vi "prepare droplet.vi"(3 "channel":i8) -> ()   [LabVIEW 2023]
panel:
  out "sum":i32
  out "entry":i32
  out "stock array":string[](array[string])
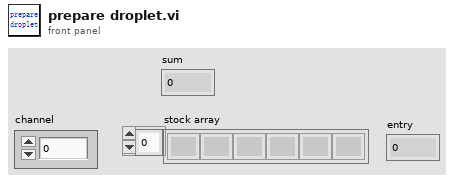
[diagram p1: front panel]
types:
  T1 = enum16{"Initialize", "Absolute Position", "Relative Pickup", "Relative Dispense", "Swich valve", "Bypass"}
  T2 = enum16{"check", "scan", "index", "read", "add", "write"}
  T3 = enum16{"plate1", "plate2", "plate3", "rinse", "seat"}
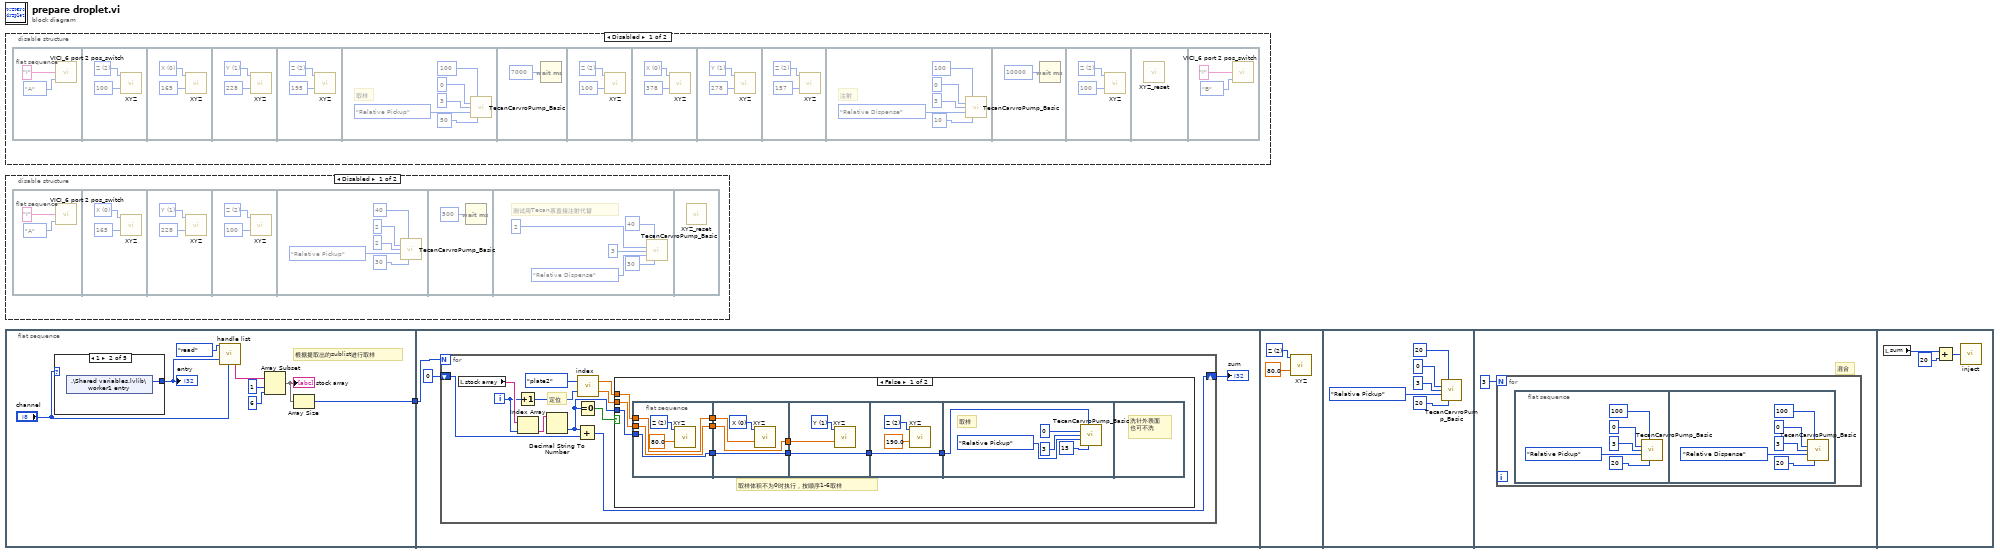
[diagram p0: block diagram]
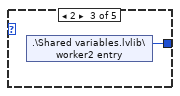
[diagram p4: hidden frame]
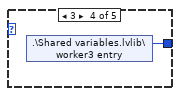
[diagram p5: hidden frame]
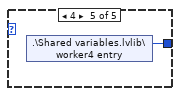
[diagram p6: hidden frame]
diagram:
  n1 = disable-structure shown="Disabled" {
    frame Disabled {
      n2 = flat-sequence {
        frame #0 {
          n3 = call "VICI_6 port 2 pos_switch.vi"("Switch to position (A/B)"=enum16{"A", "B"}."A", "Valve ID"="I") -> ()  [unwired: 2 in, 1 out]
        }
        frame #1 {
          w5 = u16 2 items=["X", "Y", "Z"] ("AXIS")
          n4 = call "XYZ.vi"("AXIS"=w5, "Set location (mm)"=100) -> ()  [unwired: 9 in, 5 out]
        }
        frame #2 {
          w7 = u16 0 items=["X", "Y", "Z"] ("AXIS")
          n5 = call "XYZ.vi"("AXIS"=w7, "Set location (mm)"=165) -> ()  [unwired: 9 in, 5 out]
        }
        frame #3 {
          w8 = u16 1 items=["X", "Y", "Z"] ("AXIS")
          n6 = call "XYZ.vi"("AXIS"=w8, "Set location (mm)"=228) -> ()  [unwired: 9 in, 5 out]
        }
        frame #4 {
          w10 = u16 2 items=["X", "Y", "Z"] ("AXIS")
          n7 = call "XYZ.vi"("AXIS"=w10, "Set location (mm)"=195) -> ()  [unwired: 9 in, 5 out]
        }
        frame #5 {
          # "取样"
          n8 = call "TecanCarvroPump_Basic.vi"("Volume (μL)"=u16 100, "TecanPump address"=u8 0, "Valve"=u8 3, "Mode"=T1."Relative Pickup", "Speed (μL/s)"=u16 50) -> ()  [unwired: 10 in, 1 out]
        }
        frame #6 {
          n9 = Wait (ms)(milliseconds to wait=u32 7000) -> ()  [unwired: 1 out]
        }
        frame #7 {
          w19 = u16 2 items=["X", "Y", "Z"] ("AXIS")
          n10 = call "XYZ.vi"("AXIS"=w19, "Set location (mm)"=100) -> ()  [unwired: 9 in, 5 out]
        }
        frame #8 {
          w20 = u16 0 items=["X", "Y", "Z"] ("AXIS")
          n11 = call "XYZ.vi"("AXIS"=w20, "Set location (mm)"=378) -> ()  [unwired: 9 in, 5 out]
        }
        frame #9 {
          w23 = u16 1 items=["X", "Y", "Z"] ("AXIS")
          n12 = call "XYZ.vi"("AXIS"=w23, "Set location (mm)"=278) -> ()  [unwired: 9 in, 5 out]
        }
        frame #10 {
          w24 = u16 2 items=["X", "Y", "Z"] ("AXIS")
          n13 = call "XYZ.vi"("AXIS"=w24, "Set location (mm)"=157) -> ()  [unwired: 9 in, 5 out]
        }
        frame #11 {
          # "注射"
          n14 = call "TecanCarvroPump_Basic.vi"("Volume (μL)"=u16 100, "TecanPump address"=u8 0, "Valve"=u8 3, "Mode"=T1."Relative Dispense", "Speed (μL/s)"=u16 10) -> ()  [unwired: 10 in, 1 out]
        }
        frame #12 {
          n15 = Wait (ms)(milliseconds to wait=u32 10000) -> ()  [unwired: 1 out]
        }
        frame #13 {
          w33 = u16 2 items=["X", "Y", "Z"] ("AXIS")
          n16 = call "XYZ.vi"("AXIS"=w33, "Set location (mm)"=100) -> ()  [unwired: 9 in, 5 out]
        }
        frame #14 {
          n17 = call "XYZ_reset.vi"() -> ()  [unwired: 12 in]
        }
        frame #15 {
          n18 = call "VICI_6 port 2 pos_switch.vi"("Switch to position (A/B)"=enum16{"A", "B"}."B", "Valve ID"="I") -> ()  [unwired: 2 in, 1 out]
        }
      }
    }
    frame Enabled {
    }
  }
  n19 = disable-structure shown="Disabled" {
    frame Disabled {
      n20 = flat-sequence {
        frame #0 {
          n21 = call "VICI_6 port 2 pos_switch.vi"("Switch to position (A/B)"=enum16{"A", "B"}."A", "Valve ID"="I") -> ()  [unwired: 2 in, 1 out]
        }
        frame #1 {
          w38 = u16 0 items=["X", "Y", "Z"] ("AXIS")
          n22 = call "XYZ.vi"("AXIS"=w38, "Set location (mm)"=165) -> ()  [unwired: 9 in, 5 out]
        }
        frame #2 {
          w41 = u16 1 items=["X", "Y", "Z"] ("AXIS")
          n23 = call "XYZ.vi"("AXIS"=w41, "Set location (mm)"=228) -> ()  [unwired: 9 in, 5 out]
        }
        frame #3 {
          w43 = u16 2 items=["X", "Y", "Z"] ("AXIS")
          n24 = call "XYZ.vi"("AXIS"=w43, "Set location (mm)"=100) -> ()  [unwired: 9 in, 5 out]
        }
        frame #4 {
          n25 = call "TecanCarvroPump_Basic.vi"("Volume (μL)"=u16 40, "TecanPump address"=u8 2, "Valve"=u8 2, "Mode"=T1."Relative Pickup", "Speed (μL/s)"=u16 30) -> ()  [unwired: 10 in, 1 out]
        }
        frame #5 {
          n26 = Wait (ms)(milliseconds to wait=u32 500) -> ()  [unwired: 1 out]
        }
        frame #6 {
          # "测试用Tecan泵直接注射代替"
          n27 = call "TecanCarvroPump_Basic.vi"("Volume (μL)"=u16 40, "TecanPump address"=u8 2, "Valve"=u8 3, "Mode"=T1."Relative Dispense", "Speed (μL/s)"=u16 30) -> ()  [unwired: 10 in, 1 out]
        }
        frame #7 {
          n28 = call "XYZ_reset.vi"() -> ()  [unwired: 12 in]
        }
      }
    }
    frame Enabled {
    }
  }
  n29 = flat-sequence {
    tunnel: [w59] -> w1
    tunnel: w1 -> [w69]
    frame #0 {
      # "根据提取出的sublist进行取样"
      n30 = case shown="1" "channel" {
        tunnel: [_ w63 w64 w65 w66] -> w55
        frame 0, Default {
        }
        frame 1 {
          n31 = shared-variable ".\\Shared variables.lvlib\\worker1 entry"() -> (w63:i32)  [unwired: 1 in, 1 out]
        }
        frame 2 {
          n32 = shared-variable ".\\Shared variables.lvlib\\worker2 entry"() -> (w64:i32)  [unwired: 1 in, 1 out]
        }
        frame 3 {
          n33 = shared-variable ".\\Shared variables.lvlib\\worker3 entry"() -> (w65:i32)  [unwired: 1 in, 1 out]
        }
        frame 4 {
          n34 = shared-variable ".\\Shared variables.lvlib\\worker4 entry"() -> (w66:i32)  [unwired: 1 in, 1 out]
        }
      }
      "entry" <- w55
      n35 = call "handle list.vi"("operation"=T2."read", "input entry"=w55, "channel"="channel") -> ("subarray"=w58:string[])  [unwired: 13 in, 3 out]
      n36 = Array Subset(array=w58, index=1, length=6) -> (w60:string[])
      "stock array" <- w60
      n37 = Array Size(array=w60) -> (size(s)=w59:i32)
    }
    frame #1 {
      n38 = for {
        N: w69 -> [_]
        shift-right: [w71] -> w67
        shift-left: 0 -> [w70]
        i -> [w77]
        # "定位"
        n39 = local read "stock array"() -> (w79:string[])
        n40 = Increment(x=w77) -> (x+1=w74:i32)
        n41 = Index Array(array=w79, index=w77) -> (element=w80:string)
        n42 = Decimal String To Number(string=w80) -> (number=w72:i32)  [unwired: 2 in, 1 out]
        n43 = Add(x=w72, y=w70) -> (x+y=w71:i32)
        n44 = Equal To 0?(x=w72) -> (x = 0?=w78:bool)
        n45 = call "index.vi"("index"=w74, "where"=T3."plate2") -> ("Y"=w75:dbl, "X"=w76:dbl)
        n46 = case shown="False" w78 {
          tunnel: w72 -> [w81 _]
          tunnel: w76 -> [w90 _]
          tunnel: w75 -> [w89 _]
          frame False {
            # "取样体积不为0时执行，按顺序1-6取样"
            n47 = flat-sequence {
              tunnel: [w93] -> w88
              tunnel: [w91] -> w87
              tunnel: [w92] -> w86
              tunnel: w90 -> [w93]
              tunnel: w81 -> [w92]
              tunnel: w89 -> [w91]
              tunnel: w88 -> [w98]
              tunnel: [w97] -> w85
              tunnel: w87 -> [w97]
              tunnel: [w96] -> w84
              tunnel: w86 -> [w96]
              tunnel: w85 -> [w101]
              tunnel: [w100] -> w83
              tunnel: w84 -> [w100]
              tunnel: w83 -> [w105]
              tunnel: [w105] -> w82
              tunnel: w82 -> [w106]
              frame #0 {
                w95 = u16 2 items=["X", "Y", "Z"] ("AXIS")
                n48 = call "XYZ.vi"("AXIS"=w95, "Set location (mm)"=80.0) -> ()  [unwired: 9 in, 5 out]
              }
              frame #1 {
                w99 = u16 0 items=["X", "Y", "Z"] ("AXIS")
                n49 = call "XYZ.vi"("AXIS"=w99, "Set location (mm)"=w98) -> ()  [unwired: 9 in, 5 out]
              }
              frame #2 {
                w102 = u16 1 items=["X", "Y", "Z"] ("AXIS")
                n50 = call "XYZ.vi"("AXIS"=w102, "Set location (mm)"=w101) -> ()  [unwired: 9 in, 5 out]
              }
              frame #3 {
                w103 = u16 2 items=["X", "Y", "Z"] ("AXIS")
                n51 = call "XYZ.vi"("AXIS"=w103, "Set location (mm)"=190.0) -> ()  [unwired: 9 in, 5 out]
              }
              frame #4 {
                # "取样"
                n52 = call "TecanCarvroPump_Basic.vi"("Volume (μL)"=w106, "TecanPump address"=u8 0, "Valve"=u8 3, "Mode"=T1."Relative Pickup", "Speed (μL/s)"=u16 15) -> ()  [unwired: 10 in, 1 out]
              }
              frame #5 {
                # "洗针外表面\n也可不洗"
              }
            }
          }
          frame True {
          }
        }
      }
      "sum" <- w67
    }
    frame #2 {
      w112 = u16 2 items=["X", "Y", "Z"] ("AXIS")
      n53 = call "XYZ.vi"("AXIS"=w112, "Set location (mm)"=80.0) -> ()  [unwired: 9 in, 5 out]
    }
    frame #3 {
      n54 = call "TecanCarvroPump_Basic.vi"("Volume (μL)"=u16 20, "TecanPump address"=u8 0, "Valve"=u8 3, "Mode"=T1."Relative Pickup", "Speed (μL/s)"=u16 20) -> ()  [unwired: 10 in, 1 out]
    }
    frame #4 {
      # "混合"
      n55 = for {
        N: 3 -> [_]
        n56 = flat-sequence {
          frame #0 {
            n57 = call "TecanCarvroPump_Basic.vi"("Volume (μL)"=u16 100, "TecanPump address"=u8 0, "Valve"=u8 3, "Mode"=T1."Relative Pickup", "Speed (μL/s)"=u16 20) -> ()  [unwired: 10 in, 1 out]
          }
          frame #1 {
            n58 = call "TecanCarvroPump_Basic.vi"("Volume (μL)"=u16 100, "TecanPump address"=u8 0, "Valve"=u8 3, "Mode"=T1."Relative Dispense", "Speed (μL/s)"=u16 20) -> ()  [unwired: 10 in, 1 out]
          }
        }
      }
    }
    frame #5 {
      n59 = local read "sum"() -> (w131:i32)
      n60 = Add(x=w131, y=20) -> (x+y=w129:i32)
      n61 = call "inject.vi"("volume"=w129) -> ()  [unwired: 1 in]
    }
  }
